vi "Epoxy Cycle Plus One.vi"(8 "error in (no error)":errorcluster, 10 "Valves Control":T2, 11 "Data Cluster In in":T1) -> (0 "error out":errorcluster, 3 "Data Cluster In out":T1)   [LabVIEW 2020]
uses:
  controls/Valves Radio.ctl
  DAQLoop_Typedef.ctl
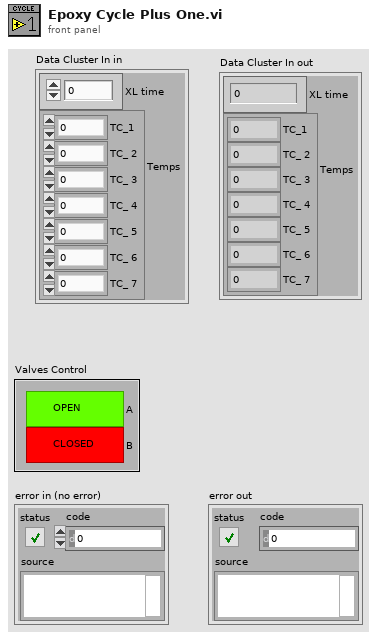
[diagram p1: front panel]
types:
  T1 = typedef "DAQLoop_Typedef.ctl" = cluster{"XL time":dbl, "Temps":cluster{"TC_1":dbl, "TC_ 2":dbl, "TC_ 3":dbl, "TC_ 4":dbl, "TC_ 5":dbl, "TC_ 6":dbl, "TC_ 7":dbl}}
  T2 = typedef "Valves Radio.ctl" = enum32{"A", "B"}
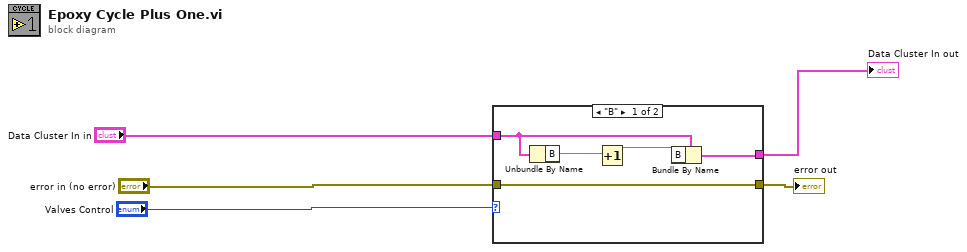
[diagram p0: block diagram]
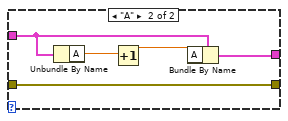
[diagram p2: hidden frame]
diagram:
  n1 = case shown="\"B\"" "Valves Control" {
    tunnel: "Data Cluster In in" -> [w6 w13]
    tunnel: [w10 w15] -> w2
    tunnel: "error in (no error)" -> [w9 w14]
    tunnel: [w9 w14] -> w4
    frame "B" {
      n2 = Unbundle By Name(w6) -> ("B"=w8:dbl)
      n3 = Increment(x=w8) -> (x+1=w7:dbl)
      n4 = Bundle By Name(cluster=w6, "B"=w7) -> (w10:T1)
    }
    frame "A" {
      n5 = Unbundle By Name(w13) -> ("A"=w12:dbl)
      n6 = Increment(x=w12) -> (x+1=w11:dbl)
      n7 = Bundle By Name(cluster=w13, "A"=w11) -> (w15:T1)
    }
  }
  "error out" <- w4
  "Data Cluster In out" <- w2
